vi "Cache_Path Global_Write.vi"(8 "error in (no error)":errorcluster, 11 "Cache Path":path) -> (0 "error out":errorcluster, 1 "Success?":bool, 3 "Non-unique Class Names":string[](array[string]))   [LabVIEW 2020, in "ClassLoader.lvlib"]
uses:
  ClassLoader.lvlib
  <vilib>/Utility/config.llb/NI_LVConfig.lvlib
  Cache_Path Global.vi
  <vilib>/Utility/config.llb/Read Key (String).vi
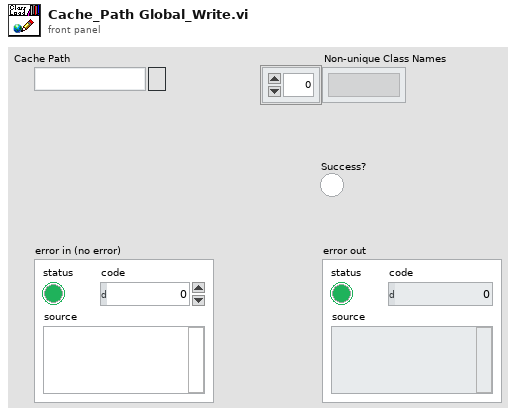
[diagram p1: front panel]
types:
  T1 = typedef "NI_LVConfig.lvlib/Config Data RefNum.ctl" = refnum<k1>
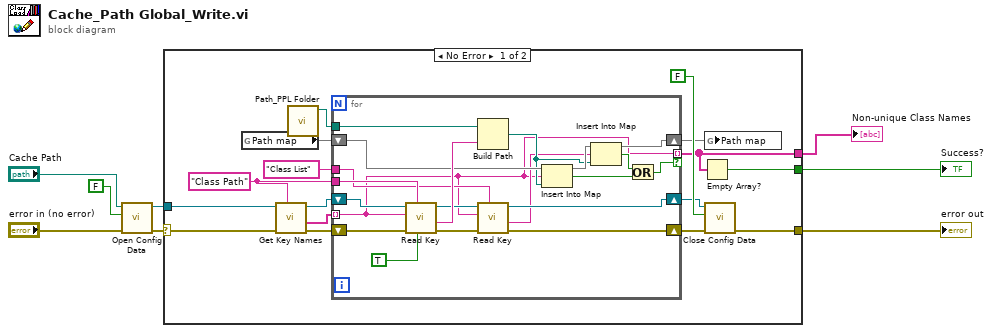
[diagram p0: block diagram]
diagram:
  n1 = call <vilib>:"Open Config Data.vi"("error in (no error)"="error in (no error)", "create file if necessary (T)"=FALSE, "configuration file path"="Cache Path") -> ("error out"=w5:errorcluster, "refnum"=w3:T1)  [unwired: 6 in, 1 out]
  n2 = case shown="No Error" w5 {
    selector: w5 -> [w22 w45]
    tunnel: [w12 w45] -> w4
    tunnel: w3 -> [w23 _]
    tunnel: [w11 _] -> w2
    tunnel: [w10 _] -> w1
    frame No Error {
      w19 = "Class Path" ("section")
      n3 = global read "Cache_Path Global.vi" "Path map"() -> (w17:map{string, path})
      n4 = call <vilib>:"Get Key Names.vi"("section"=w19, "error in (no error)"=w22, "refnum"=w23) -> ("error out"=w15:errorcluster, "key names"=w20:string[], "refnum out"=w21:T1)  [unwired: 5 in, 1 out]
      n5 = call "Path_PPL Folder.vi"() -> ("Data Folder Path"=w18:path)  [unwired: 10 in, 1 out]
      n6 = for {
        tunnel: w20 -> [w26] mode=indexing
        tunnel: w19 -> [w42]
        tunnel: w18 -> [w41]
        shift-right: [w31] -> w9
        shift-left: w17 -> [w33]
        tunnel: "Class List" ("section") -> [w39]
        shift-right: [w35] -> w13
        shift-left: w15 -> [w37]
        shift-right: [w34] -> w14
        shift-left: w21 -> [w43]
        tunnel: [w26] -> w11 mode=indexing if=w25
        n7 = call-poly <vilib>:"Read Key.vi"("read raw string? (F)"=TRUE, "section"=w42, "error in (no error)"=w37, "key"=w26, "refnum"=w43) -> ("error out"=w36:errorcluster, "value"=w40:string, "refnum out"=w38:T1)  [unwired: 3 in, 1 out]
        n8 = Build Path(base path=w41, name or relative path=w40) -> (appended path=w30:path)
        n9 = call-poly <vilib>:"Read Key.vi"("section"=w39, "error in (no error)"=w36, "key"=w26, "refnum"=w38) -> ("error out"=w35:errorcluster, "value"=w27:string, "refnum out"=w34:T1)  [unwired: 4 in, 1 out]
        n10 = Insert Into Map(map in=w33, key=w26, value=w30) -> (map out=w32:map{string, path}, key already included?=w28:bool)  [unwired: 1 out]
        n11 = Insert Into Map(map in=w32, key=w27, value=w30) -> (map out=w31:map{string, path}, key already included?=w29:bool)  [unwired: 1 out]
        n12 = Or(x=w29, y=w28) -> (x .or. y?=w25:bool)
      }
      n13 = Empty Array?(array=w11) -> (empty?=w10:bool)
      n14 = global write "Cache_Path Global.vi" "Path map"(w9) -> ()
      n15 = call <vilib>:"Close Config Data.vi"("error in (no error)"=w13, "write file if changed (T)"=FALSE, "refnum"=w14) -> ("error out"=w12:errorcluster)  [unwired: 7 in, 1 out]
    }
    frame Error {
    }
  }
  "error out" <- w4
  "Non-unique Class Names" <- w2
  "Success?" <- w1
